vi "update.vi"(7 "Pressure":dbl, 8 "error in (no error)":errorcluster, 9 "Humidity":dbl, 10 "Temperature":dbl, 11 "Observer.lvclass":refnum<class "Observer.lvclass">) -> (0 "error out":errorcluster, 3 "Observer.lvclass 2":refnum<class "Observer.lvclass">)   [LabVIEW 2020, in "Observer.lvclass"]
uses:
  Observer.lvclass
panel:
  # "Connector Pane"
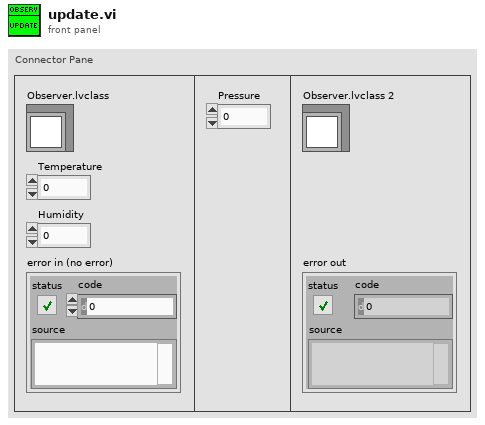
[diagram p1: front panel]
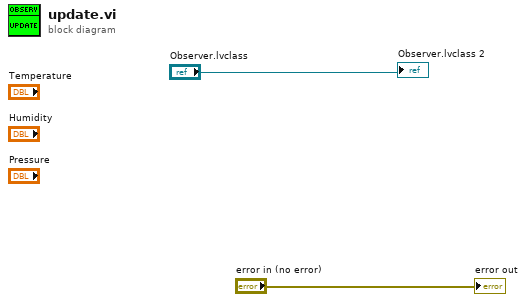
[diagram p0: block diagram]
diagram:
  "Observer.lvclass 2" <- "Observer.lvclass"
  "error out" <- "error in (no error)"
